vi "getMeasurement.vi"(7 "Source":string, 8 "error in (no error)":errorcluster, 10 "Measurement":T1=enum."Voltage Peak-Peak", 11 "Scope in":refnum<class "Scope.lvclass">) -> (0 "error out":errorcluster, 2 "Result":dbl, 3 "Scope out":refnum<class "Scope.lvclass">)   [LabVIEW 2023, in "sweScope.lvlib" / "Scope.lvclass"]
doc: "<b>Author:</b> Wolfgang\n<b>Description:</b> returns a measurement"
uses:
  Scope.lvclass
  Data/scopeMeasurements.ctl
  sweScope.lvlib
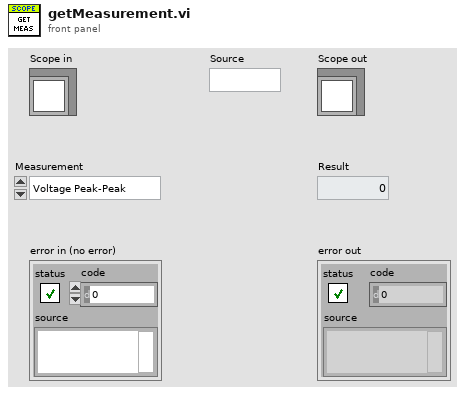
[diagram p1: front panel]
types:
  T1 = typedef "sweScope.lvlib/scopeMeasurements.ctl" = enum16{"Disable", "Mean", "Voltage Peak-Peak", "Frequency", "Amplitude", "Period", "Falling Slew Rate", "Rising Slew Rate"}
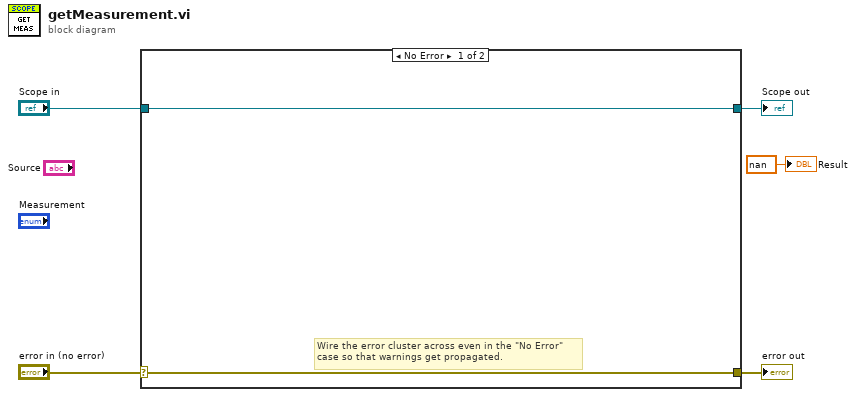
[diagram p0: block diagram]
diagram:
  n1 = case shown="No Error" "error in (no error)" {
    selector: "error in (no error)" -> [w6 w9]
    tunnel: [w6 w9] -> w4
    tunnel: [w7 w8] -> w2
    tunnel: "Scope in" -> [w7 w8]
    frame No Error {
      # "Wire the error cluster across even in the \"No Error\"\ncase so that warnings get propagated."
    }
    frame Error {
    }
  }
  "error out" <- w4
  "Scope out" <- w2
  "Result" <- nan ("Result")
